vi "DFD Probe Check Freq Response.vi"(1 "filter out":T4={"mSRate_Fs"=0.0, "mSRate_Version"="", "mSRate_Comments"="", "mSRate_OrgCoef"={"type"=enum."Undefined", "gain"=1.0, "coef a (k)"=[], "coef b (v)"=[]}, "mSRate_CurCoef"={"type"=enum."Undefined", "gain"=1.0, "coef a (k)"=[], "coef b (v)"=[]}, "mSRate_Quantized?"=FALSE, "mSRate_QCoef"={"type"=enum."Undefined", "gain"=0.0, "coef a (k)"=[], "coef b (v)"=[]}, "mSRate_QSettings"=[], "mSRate_Order"=0, "mSRate_Scaling"={"mSRate_ScaleByPowerOf2?"=FALSE, "mSRate_ScaleType"=enum."No Norm"}} {"mSRate_QSettings"."source" items=["Coef a/k"=0, "Coef b/v"=7, "Input"=1, "Output"=2, "Multiplicand"=3, "Product"=4, "Sum"=5, "Delay"=6, "Gain"=8]}) -> (0 "Boolean":bool)   [LabVIEW 2017, in "NI_DigFilterLicensed.lvlib"]
uses:
  <vilib>/addons/Digital Filter Design/NI_DigFilterLicensed.lvlib
  <vilib>/addons/Digital Filter Design/_Objects.llb/DFD Filter Obj.ctl
  <vilib>/addons/Digital Filter Design/_Objects.llb/DFD Filter Coef.ctl
  <vilib>/addons/Digital Filter Design/_Objects.llb/DFD Filter Structure Type Selector.ctl
  <vilib>/addons/Digital Filter Design/_Objects.llb/dfd_Internal Quantization Settings.ctl
  <vilib>/addons/Digital Filter Design/_Objects.llb/dfd_Internal Quantization Srcs.ctl
  <vilib>/addons/Digital Filter Design/_Objects.llb/DFD Coef Norm Type.ctl
  <vilib>/addons/Digital Filter Design/_Objects.llb/DFD Pole-Zero Plot.ctl
  <vilib>/addons/Digital Filter Design/Analysis.llb/DFD Plot Freq Response (Linear-Spaced).vi
panel:
  in  "Show Floating-Point":bool=TRUE
  in  "Show Fixed-Point":bool=TRUE
  in  "Tab Control":T1(tab)
  out "Filter Structure":u16(ring) items=["Invalid Filter", "FIR Direct Form", "FIR Direct Form Transposed", "FIR Symmetric", "FIR Antisymmetric", "IIR Direct Form I", "IIR Direct Form I Transposed", "IIR Direct Form II", "IIR Direct Form II Transposed", "IIR Cascaded Second-Order Sections I", "IIR Cascaded Second-Order Sections I Transposed", "IIR Cascaded Second-Order Sections II", "IIR Cascaded Second-Order Sections II Transposed", "Lattice Allpass (basic sections)", "Lattice Allpass (one multiplier sections)", "Lattice Allpass (normalized sections)", "Lattice AR (basic sections)", "Lattice AR (one multiplier sections)", "Lattice AR (normalized sections)", "Lattice MA (minimum phase)", "Lattice MA (maximum phase)", "Lattice ARMA (basic sections)", "Lattice ARMA (one multiplier sections)", "Lattice ARMA (normalized sections)"]
  out "Filter Order":i32=-1
  out "Quantized?":bool
  in  "dB on":bool=TRUE
  out "Magnitude":cluster{"f0":dbl, "df":dbl, "magnitude":dbl[]}[](graph)
  in  "Unwrap phase":bool=TRUE
  in  "Unit in degree":bool
  out "Phase":cluster{"f0":dbl, "df":dbl, "phase":dbl[]}[](graph)
  out "Group Delay":T2(graph)
  out "Z Plane":T3
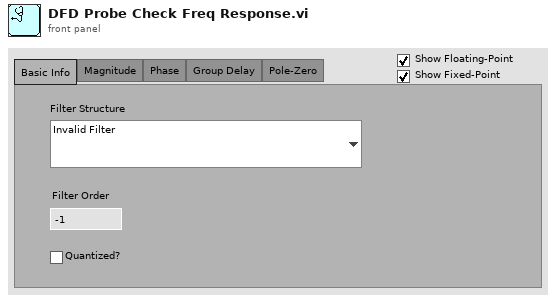
[diagram p1: front panel]
types:
  T1 = enum32{"Basic Info", "Magnitude", "Phase", "Group Delay", "Pole-Zero"}
  T2 = cluster{"f0":dbl, "df":dbl, "group delay":dbl[]}[]
  T3 = typedef "NI_DigFilterLicensed.lvlib/DFD Pole-Zero Plot.ctl" = cluster{dbl[], dbl[]}[]
  T4 = typedef "NI_DigFilterLicensed.lvlib/DFD Filter Obj.ctl" = cluster{"mSRate_Fs":dbl, "mSRate_Version":string, "mSRate_Comments":string, "mSRate_OrgCoef":T5, "mSRate_CurCoef":T5, "mSRate_Quantized?":bool, "mSRate_QCoef":T5, "mSRate_QSettings":T7[], "mSRate_Order":i32, "mSRate_Scaling":cluster{"mSRate_ScaleByPowerOf2?":bool, "mSRate_ScaleType":T9}}
  T5 = typedef "NI_DigFilterLicensed.lvlib/DFD Filter Coef.ctl" = cluster{"type":T6, "gain":dbl, "coef a (k)":dbl[], "coef b (v)":dbl[]}
  T6 = typedef "NI_DigFilterLicensed.lvlib/DFD Filter Structure Type Selector.ctl" = enum16{"Undefined", "FIR Direct Form", "FIR Direct Form Transposed", "FIR Symmetric", "FIR Antisymmetric", "IIR Direct Form I", "IIR Direct Form I Transposed", "IIR Direct Form II", "IIR Direct Form II Transposed", "IIR Cascaded Second Order Sections Form I", "IIR Cascaded Second Order Sections Form I Transposed", "IIR Cascaded Second Order Sections Form II", "IIR Cascaded Second Order Sections Form II Transposed", "Lattice Allpass (basic sections)", "Lattice Allpass (one multiplier sections)", "Lattice Allpass (normalized sections)", "Lattice AR (basic sections)", "Lattice AR (one multiplier sections)", "Lattice AR (normalized sections)", "Lattice MA (minimum phase)", "Lattice MA (maximum phase)", "Lattice ARMA (basic sections)", "Lattice ARMA (one multiplier sections)", "Lattice ARMA (normalized sections)"}
  T7 = typedef "NI_DigFilterLicensed.lvlib/dfd_Internal Quantization Settings.ctl" = cluster{"source":T8, "wl":i16, "iwl":i16, "overflow mode":enum16{"Saturation", "Wrap"}, "rounding mode":enum16{"Nearest", "Truncation"}, "signed?":bool}
  T8 = typedef "NI_DigFilterLicensed.lvlib/dfd_Internal Quantization Srcs.ctl" = u16
  T9 = typedef "NI_DigFilterLicensed.lvlib/DFD Coef Norm Type.ctl" = enum16{"No Norm", "Time Domain 1-Norm", "Time Domain 2-Norm", "Time Domain Inf-Norm"}
  T10 = cluster{"Unwrap phase":bool, "Unit in degree":bool}
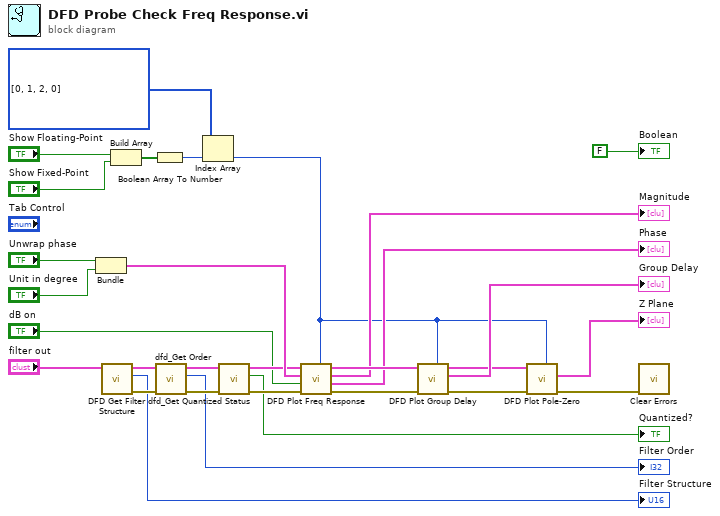
[diagram p0: block diagram]
diagram:
  w14 = u16[] [0, 1, 2, 0] items=["Auto", "Floating-point Only", "Fixed-point Only"]
  n1 = Bundle("Unwrap phase"="Unwrap phase", "Unit in degree"="Unit in degree") -> (w25:T10)  [unwired: 1 out]
  n2 = call <vilib>:"DFD Get Filter Structure.vi"("filter in"="filter out") -> ("error out"=w17:errorcluster, "structure"=→"Filter Structure":u16, "filter out"=w18:T4)  [unwired: 1 in, 7 out]
  n3 = Build Array("Show Floating-Point", "Show Fixed-Point") -> (w20:bool[])
  n4 = Boolean Array To Number(Boolean array=w20) -> (number=w19:u32)
  n5 = call <vilib>:"dfd_Get Order.vi"("error in (no error)"=w17, "filter in"=w18) -> ("error out"=w16:errorcluster, "order"=→"Filter Order":i32, "filter out"=w15:T4)  [unwired: 7 out]
  n6 = Index Array(array=w14, index=w19) -> (element=w7:u16)
  n7 = call <vilib>:"dfd_Get Quantized Status.vi"("error in (no error)"=w16, "filter in"=w15) -> ("error out"=w11:errorcluster, "quantized?"=→"Quantized?":bool, "filter out"=w12:T4)  [unwired: 7 out]
  n8 = call-poly <vilib>:"DFD Plot Freq Response.vi"("output option"=w7, "error in (no error)"=w11, "dB on? (T)"="dB on", "phase view"=w25, "filter in"=w12) -> ("error out"=w26:errorcluster, "phase response"=→"Phase":cluster{"f0":dbl, "df":dbl, "values":dbl[]}[], "magnitude response"=→"Magnitude":cluster{"f0":dbl, "df":dbl, "values":dbl[]}[], "filter out"=w28:T4)  [unwired: 3 in]
  n9 = call <vilib>:"DFD Plot Group Delay.vi"("output option"=w7, "error in (no error)"=w26, "filter in"=w28) -> ("error out"=w8:errorcluster, "group delay"=→"Group Delay":cluster{"f0":dbl, "df":dbl, "values":dbl[]}[], "filter out"=w9:T4)  [unwired: 2 in, 4 out]
  n10 = call <vilib>:"DFD Plot Pole-Zero.vi"("output option"=w7, "error in (no error)"=w8, "filter in"=w9) -> ("error out"=w5:errorcluster, "Z-Plane"=→"Z Plane":T3)  [unwired: 1 in, 6 out]
  n11 = call <vilib>:"Clear Errors.vi"("error in (no error)"=w5) -> ()  [unwired: 1 in, 6 out]
  "Boolean" <- FALSE ("Boolean")
